vi "Get Subject Parameter Folder.vi"(3 "Subject Number":u16, 4 "Create if DNE?":bool, 5 "Subject Parameter Path":path=path "Z:/CP FES Walk/2016 CP CODE/Subject_Parameters") -> (0 "Subject Number":u16, 1 "Created new?":bool, 2 "Subject Parameter Folder":path)   [LabVIEW 2019]
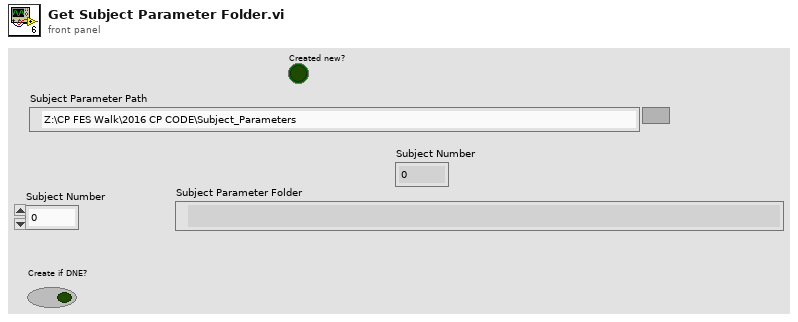
[diagram p1: front panel]
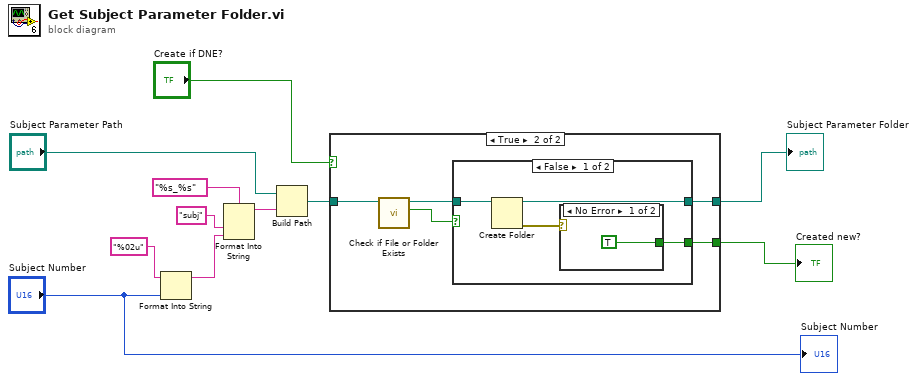
[diagram p0: block diagram]
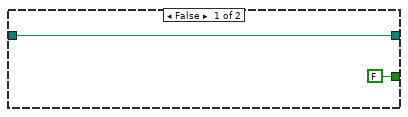
[diagram p2: hidden frame]
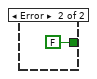
[diagram p3: hidden frame]
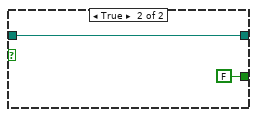
[diagram p4: hidden frame]
diagram:
  n1 = Format Into String(format string="%02u", "Subject Number") -> (resulting string=w5:string)  [unwired: 2 in, 1 out]
  n2 = Format Into String(format string="%s_%s", "subj" ("string"), w5) -> (resulting string=w7:string)  [unwired: 2 in, 1 out]
  n3 = Build Path(base path="Subject Parameter Path", name or relative path=w7) -> (appended path=w4:path)
  n4 = case shown="True" "Create if DNE?" {
    tunnel: w4 -> [w13 w18]
    tunnel: [w13 w16] -> w3
    tunnel: [FALSE w14] -> w1
    frame False {
    }
    frame True {
      n5 = call <vilib>:"Check if File or Folder Exists.vi"("path"=w18) -> ("file or folder exists?"=w15:bool, "dup path"=w17:path)  [unwired: 8 in, 1 out]
      n6 = case shown="False" w15 {
        tunnel: w17 -> [w22 w26]
        tunnel: [w21 w26] -> w16
        tunnel: [w19 FALSE] -> w14
        frame False {
          n7 = Create Folder(path (use dialog)=w22) -> (created path=w21:path, error out=w20:errorcluster)  [unwired: 2 in, 1 out]
          n8 = case shown="No Error" w20 {
            tunnel: [TRUE FALSE] -> w19
            frame No Error {
            }
            frame Error {
            }
          }
        }
        frame True {
        }
      }
    }
  }
  "Subject Parameter Folder" <- w3
  "Created new?" <- w1
  "Subject Number" <- "Subject Number"
